vi "Create.vi"(10 "error in (no error)":errorcluster, 11 "Events":T1[](array[typedef])) -> (2 "error out":errorcluster, 3 "AppStartupValue out":refnum<class "AppStartupValue.lvclass">)   [LabVIEW 2020, in "Volatus.lvlib" / "AppStartupValue.lvclass"]
uses:
  AppStartupValue.lvclass
  AppStartupValue.lvclass/AppStartupValue.ctl
  Event Level.ctl
  Volatus.lvlib
  Event.ctl
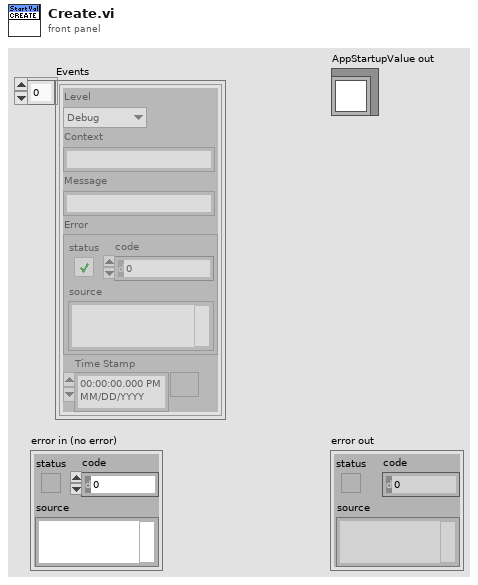
[diagram p1: front panel]
types:
  T1 = typedef "Volatus.lvlib/Event.ctl" = cluster{"Level":T2, "Context":string, "Message":string, "Error":errorcluster, "Time Stamp":timestamp}
  T2 = typedef "Volatus.lvlib/Event Level.ctl" = enum16{"Debug", "Info", "Warning", "Error"}
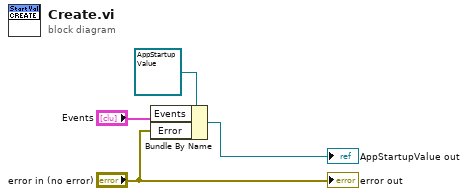
[diagram p0: block diagram]
diagram:
  n1 = Bundle By Name(cluster=refnum<class "AppStartupValue.lvclass"> refnum ("AppStartupValue in"), "Events"="Events", "Error"="error in (no error)") -> (→"AppStartupValue out":refnum<class "AppStartupValue.lvclass">)
  "error out" <- "error in (no error)"
